vi "PH_PILS.Activate Tag.vi"(0 "i ref in":refnum<vi>, 2 "Tag Name":string="N/A", 5 "error in (no error)":errorcluster) -> (14 "i ref out":refnum<vi>, 19 "error out":errorcluster)   [LabVIEW 2014, in "PH_PILS.lvlib"]
doc: "This VI sends a \"true\" to the tag, waits 250ms, and sends a \"false\" afterwards. This is meant to actice relais."
uses:
  PH_PILS.lvlib
  PH_Beckhoff/PH_Beckhoff.lvlib
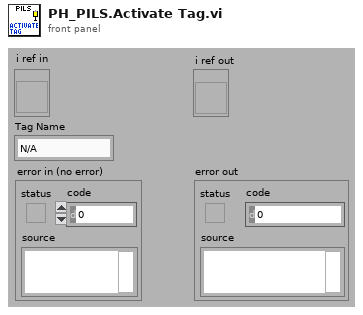
[diagram p1: front panel]
types:
  T1 = typedef "PH_PILS.lvlib/PH_PILS.i attribute.ctl" = cluster{"Boolean":cluster{"GUI Ref":refnum<vi>, "Status":i32}[], "GUI Refs Exp. Shutters":cluster{"1":refnum<vi>, "2":refnum<vi>, "3":refnum<vi>, "4":refnum<vi>}, "Tristate2Run GUI Refs":refnum<vi>[], "EO-Likes":cluster{"GUI Ref":refnum<vi>, "Status":i32}[], "Operation Mode":cluster{"Operation Mode":T2, "GUI":cluster{"Ref State":refnum<vi>, "Ref":refnum<vi>}, "Servicemode":cluster{"Tagname":string, "Status":i32}, "Labormode":cluster{"Tagname":string, "Status":i32}, "Searchmode":cluster{"Tagname":string, "Status":i32}, "Shotmode":cluster{"Tagname":string, "Status":i32}}, "Submode":cluster{"Submode":T3, "GUI":cluster{"Ref State":refnum<vi>, "Ref":refnum<vi>}, "Submode":cluster{"Tagname":string, "Status":i32}}, "Experiment":cluster{"Experiment":enum16{"unknown", "intern", "4 (Z6)", "3", "2", "1"}, "GUI":cluster{"Ref State":refnum<vi>, "Ref":refnum<vi>}, "intern":cluster{"Tagname":string, "Status":i32}, "Exp 4":cluster{"Tagname":string, "Status":i32}, "Exp 3":cluster{"Tagname":string, "Status":i32}, "Exp 2":cluster{"Tagname":string, "Status":i32}, "Exp 1":cluster{"Tagname":string, "Status":i32}}, "TristateNormal":cluster{"GUI Ref":refnum<vi>, "Status":i32}[], "Door Tags":cluster{"GUI Ref":refnum<vi>, "Status":i32}[], "GUIlessTags":cluster{"Name":string, "Status":i32}[], "Beamline GUI Refs":refnum<vi>[], "Special Boolean":cluster{"GUI Ref":refnum<vi>, "Status":i32}[], "Laserpower":cluster{"GUI Ref":refnum<vi>, "Status":i32}[], "Shutter":cluster{"GUI Ref":refnum<vi>, "Status":i32}[], "Tristate EO Like":cluster{"GUI Ref":refnum<vi>, "Status":i32}[], "PP":cluster{"GUI Ref":refnum<vi>, "Status":i32, "Head Ref":refnum<vi>, "Slider Ref":refnum<vi>}[], "Switch Knobs":cluster{"GUI Ref":refnum<vi>, "Status":i32}[], "Latch Knob GUI Refs":refnum<vi>[], "FailureCounter":i32, "Enabled Status":cluster{"Laser":i32, "PreAmp":i32, "MainAmp":i32}, "Mercury":refnum<vi>, "Instance Rods":string, "Logfile":path, "Beckhoff-Instance Internal":string, "Beckhoff-Instance External":string, "Enabling Rights":cluster{"Name":string, "Password":string, "PA?":bool, "MA?":bool, "Exp?":bool}[]}
  T2 = typedef "PH_PILS.lvlib/PH_PILS.Operation Mode.ctl" = enum16{"unknown", "Service", "Labor", "Search", "Shot"}
  T3 = typedef "PH_PILS.lvlib/PH_PILS.Submode.ctl" = enum16{"unknown", "HV-Normal", "HV-Test"}
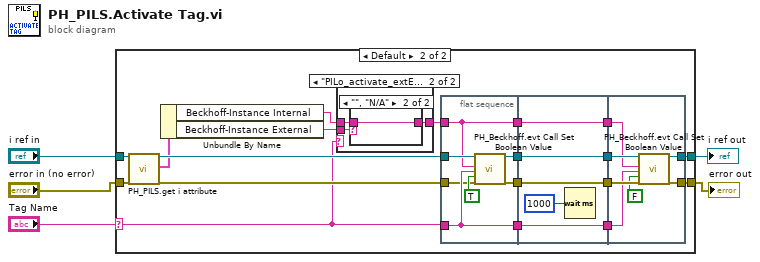
[diagram p0: block diagram]
diagram:
  n1 = case shown="Default" "Tag Name" {
    selector: "Tag Name" -> [_ w12]
    tunnel: "i ref in" -> [w7 w14]
    tunnel: "error in (no error)" -> [w6 w18]
    tunnel: [w6 w20] -> w3
    tunnel: [w7 w19] -> w2
    frame "", "N/A" {
    }
    frame Default {
      n2 = call "PH_PILS.get i attribute.vi"("i ref in"=w14, "error in (no error)"=w18) -> ("i ref out"=w13:refnum<vi>, "i attribute"=w10:T1, "error out"=w15:errorcluster)  [unwired: 15 in]
      n3 = Unbundle By Name(w10) -> ("Beckhoff-Instance Internal"=w9:string, "Beckhoff-Instance External"=w8:string)
      n4 = case shown="\"PILo_activate_extEmergencies\", \"PILo_enable_exp1\", \"PILo_enable_exp2\", \"PILo_enable_exp3\", \"PILo_enable_exp4\"" w12 {
        tunnel: w8 -> [_ w30]
        tunnel: w9 -> [w27 w29]
        tunnel: [w27 w28] -> w11
        frame Default {
        }
        frame "PILo_activate_extEmergencies", "PILo_enable_exp1", "PILo_enable_exp2", "PILo_enable_exp3", "PILo_enable_exp4" {
          n5 = case shown="\"\", \"N/A\"" w30 {
            selector: w30 -> [w31 _]
            tunnel: [w31 w32] -> w28
            tunnel: w29 -> [_ w32]
            frame Default {
            }
            frame "", "N/A" {
            }
          }
        }
      }
      n6 = flat-sequence {
        tunnel: w12 -> [w36]
        tunnel: [w39] -> w26
        tunnel: [w38] -> w25
        tunnel: [w36] -> w24
        tunnel: w15 -> [w35]
        tunnel: w13 -> [w34]
        tunnel: w11 -> [w33]
        tunnel: [w33] -> w16
        tunnel: w26 -> [w44]
        tunnel: w25 -> [w43]
        tunnel: [w44] -> w23
        tunnel: [w43] -> w22
        tunnel: [w41] -> w21
        tunnel: w24 -> [w41]
        tunnel: [w40] -> w17
        tunnel: w16 -> [w40]
        tunnel: [w50] -> w19
        tunnel: [w48] -> w20
        tunnel: w23 -> [w49]
        tunnel: w22 -> [w51]
        tunnel: w21 -> [w46]
        tunnel: w17 -> [w45]
        frame #0 {
          n7 = call "PH_Beckhoff.evt Call Set Boolean Value.vi"("i ref in"=w34, "Beckhoff Instance"=w33, "Tagname to set"=w36, "Value"=TRUE ("Value to set"), "error in"=w35) -> ("i ref out"=w38:refnum<vi>, "error out"=w39:errorcluster)  [unwired: 13 in]
        }
        frame #1 {
          n8 = Wait (ms)(milliseconds to wait=u32 1000) -> ()  [unwired: 1 out]
        }
        frame #2 {
          n9 = call "PH_Beckhoff.evt Call Set Boolean Value.vi"("i ref in"=w51, "Beckhoff Instance"=w45, "Tagname to set"=w46, "Value"=FALSE ("Value to set"), "error in"=w49) -> ("i ref out"=w50:refnum<vi>, "error out"=w48:errorcluster)  [unwired: 13 in]
        }
      }
    }
  }
  "i ref out" <- w2
  "error out" <- w3
